vi "Result_Test.vi"(8 "error in (no error)":errorcluster caption="entrée d'erreur (pas d'erreur)", 11 "P1833_Access_Code.lvclass":refnum<class "P1833_Access_Code.lvclass">) -> (0 "error out":errorcluster caption="sortie d'erreur", 3 "P1833_Access_Code.lvclass":refnum<class "P1833_Access_Code.lvclass">)   [LabVIEW 2020, in "Library Test.lvlib" / "P1833_Access_Code.lvclass"]
uses:
  P1833_Access_Code.lvclass
  C:/Users/ngarcin/OneDrive - Altyor/Standard TB/Suite TB45/Class/Test/Test (Default)/Test (Default).lvclass
  Commun VI/TypeDef/Variable Printable.ctl
  Test_Without_Instr/Test_Without_Inst.lvclass
  Commun VI/Library Commun.lvlib
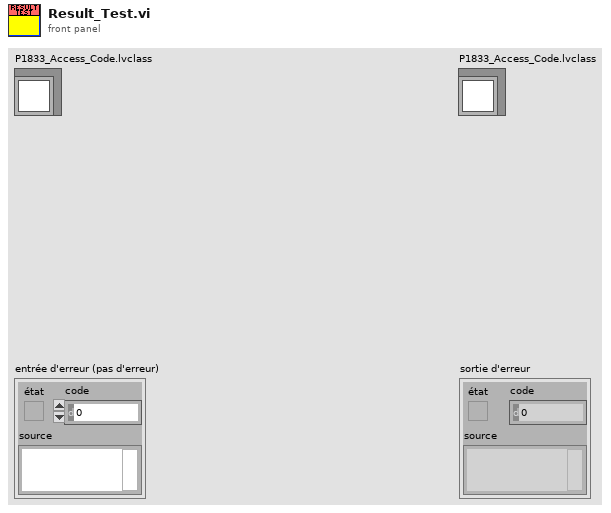
[diagram p1: front panel]
types:
  T1 = enum16{"Get Variable", "Get All Variables", "Set Variable", "Delete Variable", "Delete All Variable"}
  T2 = typedef "Variable Printable.ctl" = string
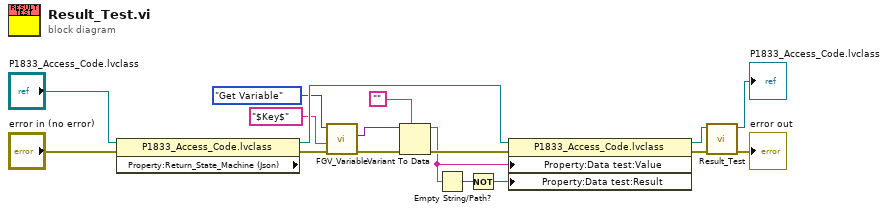
[diagram p0: block diagram]
diagram:
  n1 = property class="P1833_Access_Code.lvclass" props=["Property:Return_State_Machine (Json)"](reference="P1833_Access_Code.lvclass", error in="error in (no error)") -> (reference out=w14:refnum<class "P1833_Access_Code.lvclass">, error out=w11:errorcluster)  [unwired: 1 out]
  n2 = call "FGV_Variable.vi"("error in (no error)"=w11, "Variable"=T2 "$Key$", "Function"=T1."Get Variable") -> ("error out"=w8:errorcluster, "Data Out"=w5:variant)  [unwired: 6 in, 1 out]
  n3 = Variant To Data(error in=w8, type="", Variant=w5) -> (data=w2:string, error out=w7:errorcluster)
  n4 = Empty String/Path?(string/path=w2) -> (empty?=w4:bool)
  n5 = Not(x=w4) -> (.not. x?=w3:bool)
  n6 = property class="P1833_Access_Code.lvclass"(reference=w14, error in=w7, "Property:Data test:Value"=w2, "Property:Data test:Result"=w3) -> (reference out=w9:refnum<class "P1833_Access_Code.lvclass">, error out=w10:errorcluster)
  n7 = call-parent "Result_Test.vi"("error in (no error)"=w10, "Test_Without_Inst en entrée"=w9) -> ("error out"=→"error out":errorcluster, "Test_Without_Inst en sortie"=→"P1833_Access_Code.lvclass":refnum<class "P1833_Access_Code.lvclass">)  [unwired: 8 in]
